vi "TB-Initialize Pistonphone Measurement.vi"(0 "Exposure parameters":T1={"Low cutoff (kHz)"=8.0, "High cutoff (kHz)"=16.0, "Duration (min)"=120.0, "dB SPL"=100.0, "Waveform"=enum."Tone", "WAVfile"=path "", "refWav"=path "", "use mic correction"=FALSE, "micCorrFile"=path "", "Pistonphone Level (dB SPL)"=0.0, "Sampling rate (Hz)"=0.0, "Buffer length (s)"=0.0, "Stream mic"=FALSE, "Fine adjust"={"Max"=0.0, "Min"=0.0}, "Mic gain"=0.0, "atten"=0.0, "resol (Hz)"=0.0, "navgs"=0, "Allow Slack"=FALSE, "max starts"=0, "Freq (kHz)"=8.0, "Tma (s)"=0.0, "Streamed"=[], "Drive"="", "Speaker"="", "Mic"=""}, 11 "error in (no error)":errorcluster) -> (4 "Params thru":T1={"Low cutoff (kHz)"=8.0, "High cutoff (kHz)"=16.0, "Duration (min)"=120.0, "dB SPL"=100.0, "Waveform"=enum."Tone", "WAVfile"=path "", "refWav"=path "", "use mic correction"=FALSE, "micCorrFile"=path "", "Pistonphone Level (dB SPL)"=0.0, "Sampling rate (Hz)"=0.0, "Buffer length (s)"=0.0, "Stream mic"=FALSE, "Fine adjust"={"Max"=0.0, "Min"=0.0}, "Mic gain"=0.0, "atten"=0.0, "resol (Hz)"=0.0, "navgs"=0, "Allow Slack"=FALSE, "max starts"=0, "Freq (kHz)"=8.0, "Tma (s)"=0.0, "Streamed"=[], "Drive"="", "Speaker"="", "Mic"=""}, 15 "error out":errorcluster)   [LabVIEW 2020]
uses:
  Typedefs/TB-Parameters.ctl
  epl-vi-lib/PXI DAQ VIs/AIDI/Typedefs/AIDI-Config.ctl
  epl-vi-lib/PXI DAQ VIs/AIDI/Typedefs/AIDI-Output Spec.ctl
  epl-vi-lib/PXI DAQ VIs/AIDI/Typedefs/DI-Output Spec.ctl
  epl-vi-lib/PXI DAQ VIs/AIDI/Typedefs/AIDI-Action.ctl
panel:
  in  "T (ms)":dbl=1000.0 caption="Frame size (ms)"
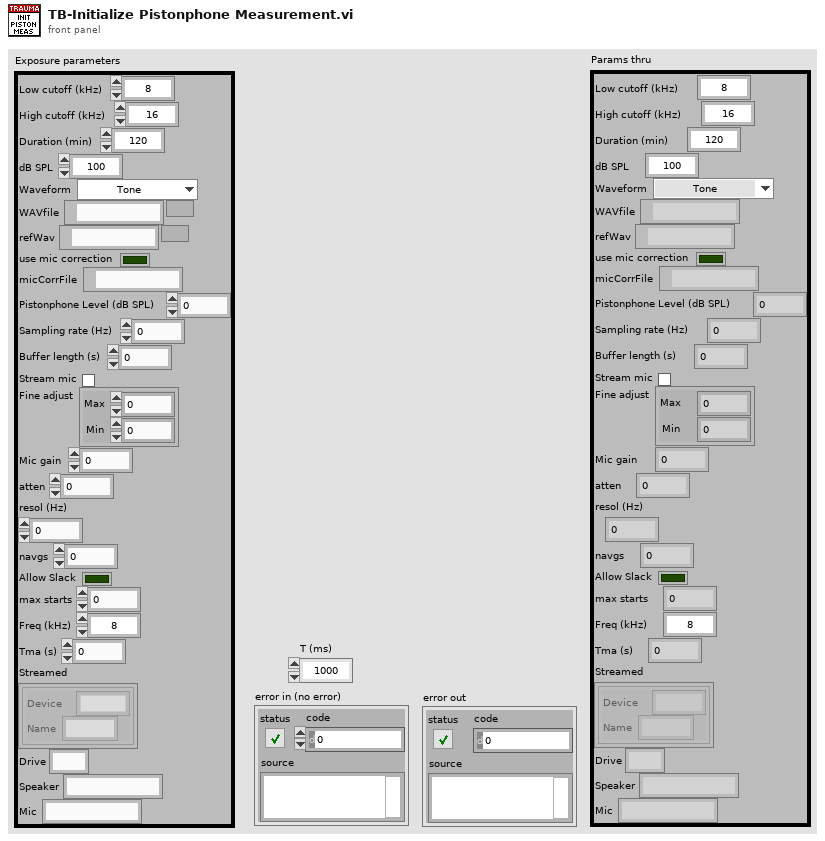
[diagram p1: front panel]
types:
  T1 = typedef "TB-Parameters.ctl" = cluster{"Low cutoff (kHz)":dbl, "High cutoff (kHz)":dbl, "Duration (min)":dbl, "dB SPL":dbl, "Waveform":enum16{"Noise", "File", "Tone"}, "WAVfile":path, "refWav":path, "use mic correction":bool, "micCorrFile":path, "Pistonphone Level (dB SPL)":dbl, "Sampling rate (Hz)":dbl, "Buffer length (s)":dbl, "Stream mic":bool, "Fine adjust":cluster{"Max":dbl, "Min":dbl}, "Mic gain":dbl, "atten":dbl, "resol (Hz)":dbl, "navgs":i32, "Allow Slack":bool, "max starts":i32, "Freq (kHz)":dbl, "Tma (s)":dbl, "Streamed":cluster{"Device":string, "Name":string}[], "Drive":string, "Speaker":string, "Mic":string}
  T2 = typedef "AIDI-Action.ctl" = enum16{"Configure", "Initialize", "Start", "Read", "Clean up", "Init & Start", "Config & Test", "Position"}
  T3 = typedef "AIDI-Config.ctl" = cluster{"AI":T4, "DI":T5, "ExtTrig":bool}
  T4 = typedef "AIDI-Output Spec.ctl" = cluster{"Channels":string[], "Fs (Hz)":dbl, "Npts":i32}
  T5 = typedef "DI-Output Spec.ctl" = cluster{"Channels":string[], "Fs (Hz)":dbl, "Npts":i32, "Port":string}
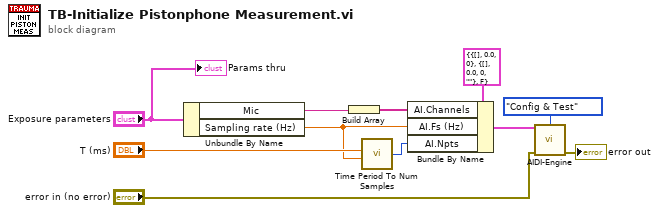
[diagram p0: block diagram]
diagram:
  n1 = Unbundle By Name("Exposure parameters") -> ("Mic"=w4:string, "Sampling rate (Hz)"=w2:dbl)
  n2 = Build Array(w4) -> (w3:string[])
  n3 = call "Time Period To Num Samples.vi"("Duration (ms)"="T (ms)", "Sampling rate (Hz)"=w2) -> ("Samples"=w11:i32)  [unwired: 5 in]
  n4 = Bundle By Name(cluster=T3 {"AI"={"Channels"=[], "Fs (Hz)"=0.0, "Npts"=0}, "DI"={"Channels"=[], "Fs (Hz)"=0.0, "Npts"=0, "Port"=""}, "ExtTrig"=FALSE} ("Config"), "AI.Channels"=w3, "AI.Fs (Hz)"=w2, "AI.Npts"=w11) -> (w7:T3)
  n5 = call "AIDI-Engine.vi"("Config"=w7, "Action"=AIDI-Action."Config & Test", "error in (no error)"="error in (no error)") -> ("error out"=→"error out":errorcluster)  [unwired: 9 in, 3 out]
  "Params thru" <- "Exposure parameters"
